vi "公式节点的使用.vi"() -> ()   [LabVIEW 2018]
panel:
  out "ans":dbl
  in  "b":dbl
  in  "a":dbl
  out "等级":dbl
  in  "考试分数":dbl
  out "y":dbl
  out "x":dbl
  in  "c":dbl
  in  "b":dbl
  in  "a":dbl
  # "1.x =a+b+c  y=a*b*c"
  # "2.if多状态判断"
  # "3.计算a*b+(a+1)*(b+1)+(a+2)*(b+2)+...+(a+999)*(b+999)"
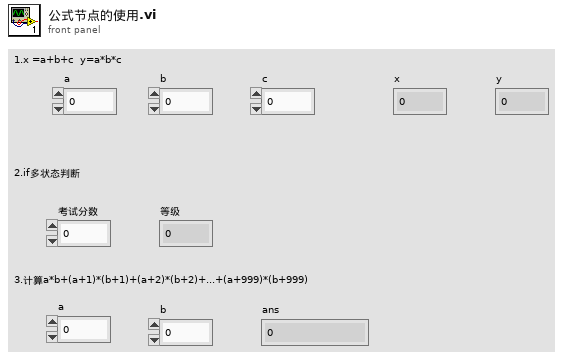
[diagram p1: front panel]
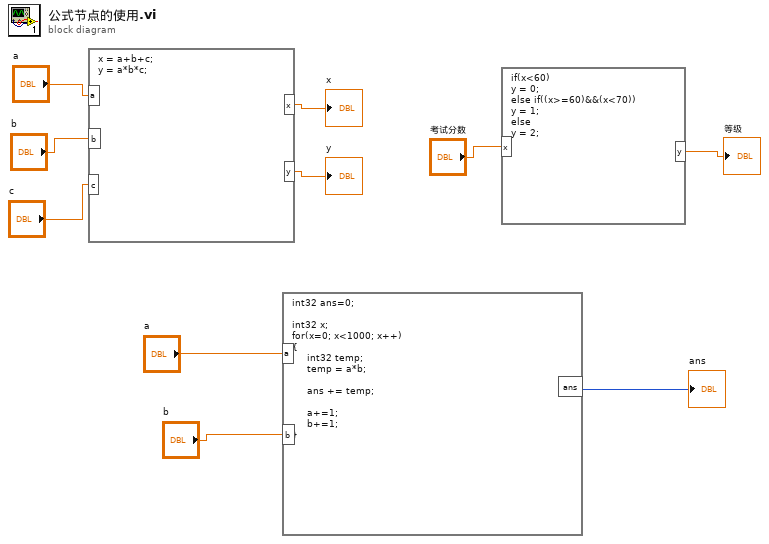
[diagram p0: block diagram]
diagram:
  n1 = formula code="x = a+b+c;\ny = a*b*c;"("a"="a", "b"="b", "c"="c") -> ("x"=→"x":dbl, "y"=→"y":dbl)
  n2 = formula code="int32 ans=0;\n\nint32 x;\nfor(x=0; x<1000; x++)\n{\n     int32 temp;\n     temp = a*b;\n     \n     ans += temp;\n\n     a+=1;\n     b+=1;\n}"("a"="a", "b"="b") -> ("ans"=→"ans":i32)
  n3 = formula code="if(x<60)\ny = 0;\nelse if((x>=60)&&(x<70))\ny = 1;\nelse\ny = 2;"("x"="考试分数") -> ("y"=→"等级":dbl)
